vi "FindMinSteerAngleError.vi"(6 "Motor Power":dbl format="%#_13g", 8 "Drive Mode":T1, 9 "Desired Angle":dbl format="%#_13g", 11 "Actual Angle":dbl format="%#_13g") -> (4 "Angle Error":dbl, 5 "Motor Power":dbl)   [LabVIEW 2019]
uses:
  Controls/Robot Drive Mode.ctl
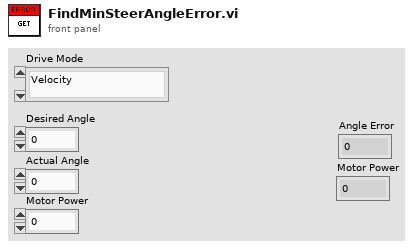
[diagram p1: front panel]
types:
  T1 = typedef "Robot Drive Mode.ctl" = enum16{"Velocity", "Distance"}
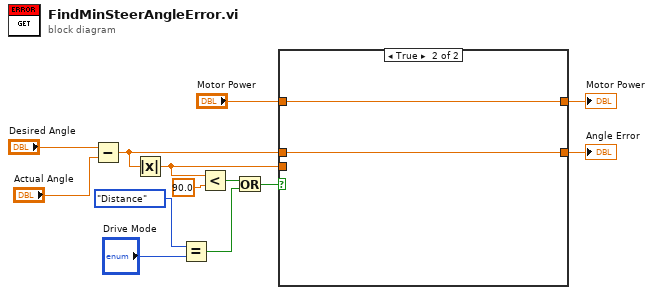
[diagram p0: block diagram]
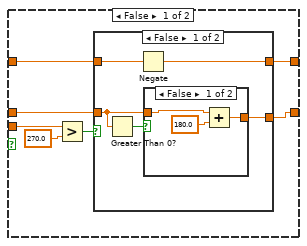
[diagram p2: hidden frame]
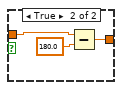
[diagram p3: hidden frame]
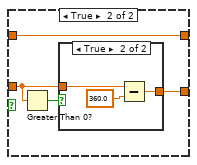
[diagram p4: hidden frame]
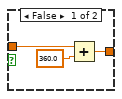
[diagram p5: hidden frame]
diagram:
  n1 = Subtract(x="Desired Angle", y="Actual Angle") -> (x-y=w10:dbl)
  n2 = Absolute Value(x=w10) -> (abs(x)=w8:dbl)
  n3 = Equal?(x=Robot_Drive_Mode."Distance" ("Drive Mode"), y="Drive Mode") -> (x = y?=w3:bool)
  n4 = Less?(x=w8, y=90.0) -> (x < y?=w2:bool)
  n5 = Or(x=w2, y=w3) -> (x .or. y?=w1:bool)
  n6 = case shown="True" w1 {
    tunnel: w10 -> [w18 w42]
    tunnel: "Motor Power" -> [w17 w43]
    tunnel: w8 -> [w20 _]
    tunnel: [w16 w43] -> w7
    tunnel: [w15 w42] -> w6
    frame False {
      n7 = Greater?(x=w20, y=270.0) -> (0:w14:bool)
      n8 = case shown="False" w14 {
        tunnel: w18 -> [w25 w34]
        tunnel: w17 -> [w23 w32]
        tunnel: [w22 w32] -> w16
        tunnel: [w21 w33] -> w15
        frame False {
          n9 = Greater Than 0?(x=w25) -> (x > 0?=w24:bool)
          n10 = Negate(x=w23) -> (-x=w22:dbl)
          n11 = case shown="False" w24 {
            tunnel: w25 -> [w28 w31]
            tunnel: [w26 w29] -> w21
            frame False {
              n12 = Add(x=w28, y=180.0) -> (x+y=w26:dbl)
            }
            frame True {
              n13 = Subtract(x=w31, y=180.0) -> (x-y=w29:dbl)
            }
          }
        }
        frame True {
          n14 = Greater Than 0?(x=w34) -> (x > 0?=w35:bool)
          n15 = case shown="True" w35 {
            tunnel: w34 -> [w38 w41]
            tunnel: [w36 w39] -> w33
            frame False {
              n16 = Add(x=w38, y=360.0) -> (x+y=w36:dbl)
            }
            frame True {
              n17 = Subtract(x=w41, y=360.0) -> (x-y=w39:dbl)
            }
          }
        }
      }
    }
    frame True {
    }
  }
  "Motor Power" <- w7
  "Angle Error" <- w6
